vi "AMZ_S3_API_Create Grantee XML String (Person ID).vi"(4 "Person ID":T1) -> (1 "Grantee":string)   [LabVIEW 2011, in "LV Interface for Amazon S3.lvlib"]
uses:
  LV Interface for Amazon S3.lvlib
  Typedefs/AMZ_S3_API_Owner.ctl
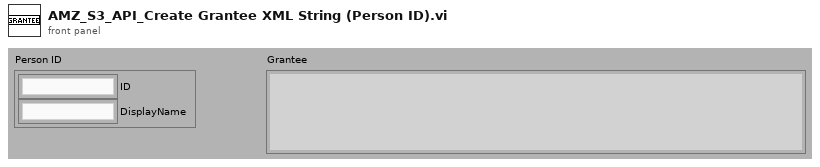
[diagram p1: front panel]
types:
  T1 = typedef "LV Interface for Amazon S3.lvlib/AMZ_S3_API_Owner.ctl" = cluster{"ID":string, "DisplayName":string}
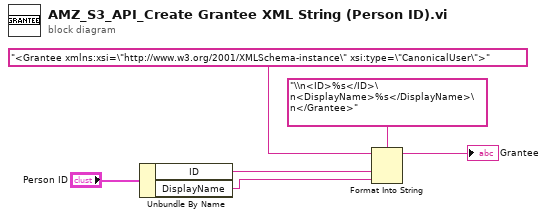
[diagram p0: block diagram]
diagram:
  n1 = Unbundle By Name("Person ID") -> ("ID"=w3:string, "DisplayName"=w2:string)
  n2 = Format Into String(format string="\\n<ID>%s</ID>\n<DisplayName>%s</DisplayName>\n</Grantee>", initial string="<Grantee xmlns:xsi=\"http://www.w3.org/2001/XMLSchema-instance\" xsi:type=\"CanonicalUser\">", w3, w2) -> (resulting string=→"Grantee":string)  [unwired: 1 in, 1 out]
